vi "setRange.vi"(8 "error in (no error)":errorcluster, 10 "range":dbl, 11 "DmmNiPxi in":refnum<class "DmmNi.lvclass">) -> (0 "error out":errorcluster, 3 "DmmNiPxi out":refnum<class "DmmNi.lvclass">)   [LabVIEW 2023, in "DmmNi.lvclass"]
doc: "<b>Author:</b> Wolfgang\n<b>Description:</b> Measurement range of the dmm based on the previously defined mode"
uses:
  DmmNi.lvclass
  DmmNi.lvclass/DmmNi.ctl
  Multimeter.lvclass
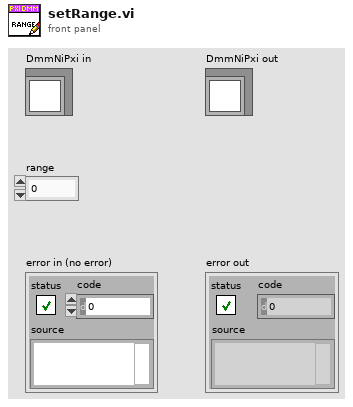
[diagram p1: front panel]
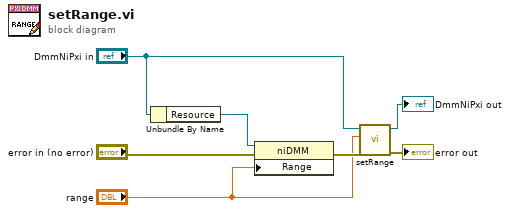
[diagram p0: block diagram]
diagram:
  n1 = Unbundle By Name("DmmNiPxi in") -> ("Resource"=w4:refnum<k15>)
  n2 = property class="niDMM"(reference=w4, error in="error in (no error)", "Range"="range") -> (error out=w3:errorcluster)  [unwired: 1 out]
  n3 = call-parent "setRange.vi"("error in (no error)"=w3, "Range"="range", "Multimeter in"="DmmNiPxi in") -> ("error out"=→"error out":errorcluster, "Multimeter out"=→"DmmNiPxi out":refnum<class "DmmNi.lvclass">)  [unwired: 7 in]
